vi "TrapezoidalMotionProfile.vi"(6 "Initialize":bool, 10 "Time":dbl, 11 "Config":T2={"TargetPos"=10.0, "InitalPos"=0.0, "FinalVel"=0.0, "IntitialVel"=0.0, "MaxVel"=10.0, "MaxAccel"=10.0}) -> (0 "Done":bool, 2 "Velocity":dbl, 3 "Distance":dbl)   [LabVIEW 2017]
panel:
  out "Data 2":T1
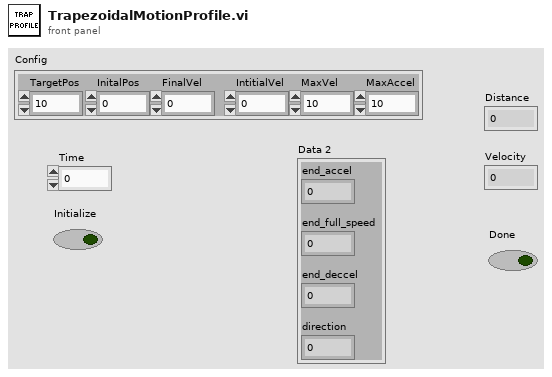
[diagram p1: front panel]
types:
  T1 = cluster{"end_accel":dbl, "end_full_speed":dbl, "end_deccel":dbl, "direction":dbl}
  T2 = cluster{"TargetPos":dbl, "InitalPos":dbl, "FinalVel":dbl, "IntitialVel":dbl, "MaxVel":dbl, "MaxAccel":dbl}
  T3 = cluster{"Config":cluster{"TargetPos":dbl, "InitalPos":dbl, "FinalVel":dbl, "IntitialVel":dbl, "MaxVel":dbl, "MaxAccel":dbl}, "Data 2":cluster{"end_accel":dbl, "end_full_speed":dbl, "end_deccel":dbl, "direction":dbl}}
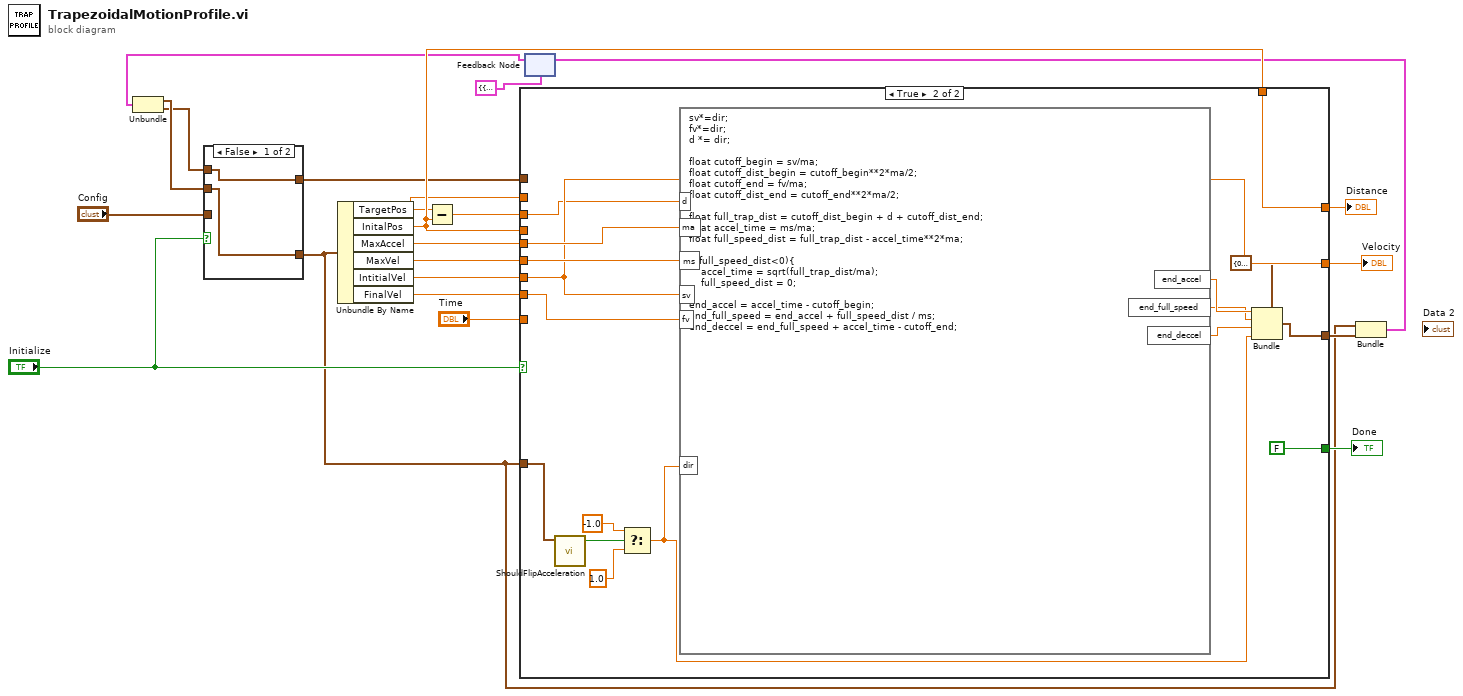
[diagram p0: block diagram]
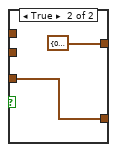
[diagram p2: hidden frame]
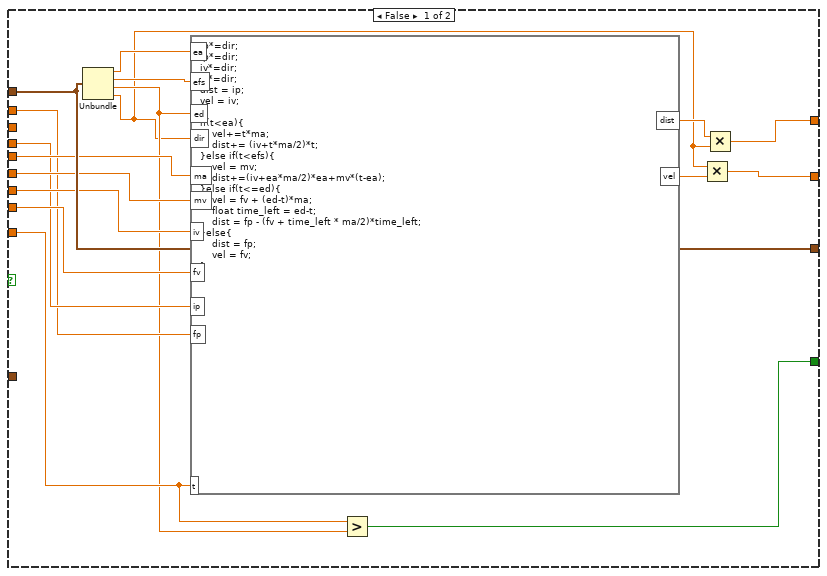
[diagram p3: hidden frame]
diagram:
  n1 = feedback #1(T3 {"Config"={"TargetPos"=10.0, "InitalPos"=0.0, "FinalVel"=0.0, "IntitialVel"=0.0, "MaxVel"=10.0, "MaxAccel"=10.0}, "Data 2"={"end_accel"=0.0, "end_full_speed"=0.0, "end_deccel"=0.0, "direction"=0.0}} ("AllData")) -> (w6:T3)
  n2 = Unbundle(w6) -> ("Config"=w5:T2, "Data 2"=w4:T1)
  n3 = case shown="False" "Initialize" {
    tunnel: [w22 T1 {"end_accel"=0.0, "end_full_speed"=0.0, "end_deccel"=0.0, "direction"=0.0} ("Data 2")] -> w9
    tunnel: [w23 w24] -> w2
    tunnel: "Config" -> [_ w24]
    tunnel: w5 -> [w23 _]
    tunnel: w4 -> [w22 _]
    frame False {
    }
    frame True {
    }
  }
  n4 = Unbundle By Name(w2) -> ("TargetPos"=w11:dbl, "InitalPos"=w12:dbl, "MaxAccel"=w21:dbl, "MaxVel"=w20:dbl, "IntitialVel"=w18:dbl, "FinalVel"=w14:dbl)
  n5 = Subtract(x=w11, y=w12) -> (x-y=w19:dbl)
  n6 = case shown="True" "Initialize" {
    tunnel: w21 -> [w39 w59]
    tunnel: w20 -> [w37 w58]
    tunnel: w18 -> [w38 w56]
    tunnel: w19 -> [_ w48]
    tunnel: [w27 w56] -> w17
    tunnel: [w29 w47] -> w13
    tunnel: w9 -> [w42 _]
    tunnel: [w42 w46] -> w3
    tunnel: "Time" -> [w33 _]
    tunnel: [w31 FALSE ("Initialize")] -> w15
    tunnel: w2 -> [_ w54]
    tunnel: w14 -> [w36 w53]
    tunnel: w12 -> [_ w47]
    tunnel: w12 -> [w35 _]
    tunnel: w11 -> [w34 _]
    frame False {
      n7 = Unbundle(w42) -> ("end_accel"=w41:dbl, "end_full_speed"=w40:dbl, "end_deccel"=w32:dbl, "direction"=w26:dbl)
      n8 = formula code="ip*=dir;\nfp*=dir;\niv*=dir;\nfv*=dir;\ndist = ip;\nvel = iv;\n\nif(t<ea){\n    vel+=t*ma;\n    dist+= (iv+t*ma/2)*t;\n}else if(t<efs){\n    vel = mv;\n    dist+=(iv+ea*ma/2)*ea+mv*(t-ea);\n}else if(t<=ed){\n    vel = fv + (ed-t)*ma;\n    float time_left = ed-t;\n    dist = fp - (fv + time_left * ma/2)*time_left;\n}else{\n    dist = fp;\n    vel = fv;\n}"("t"=w33, "ea"=w41, "efs"=w40, "ed"=w32, "ma"=w39, "iv"=w38, "mv"=w37, "fv"=w36, "ip"=w35, "fp"=w34, "dir"=w26) -> ("dist"=w30:dbl, "vel"=w28:dbl)
      n9 = Greater?(x=w33, y=w32) -> (0:w31:bool)
      n10 = Multiply(x=w26, y=w28) -> (x*y=w27:dbl)
      n11 = Multiply(x=w30, y=w26) -> (x*y=w29:dbl)
    }
    frame True {
      n12 = call "ShouldFlipAcceleration.vi"("Config"=w54) -> ("Flip?"=w51:bool)  [unwired: 10 in]
      n13 = Select(t=-1.0, s=w51, f=1.0) -> (s? t:f=w43:dbl)
      n14 = formula code="sv*=dir;\nfv*=dir;\nd *= dir;\n\nfloat cutoff_begin = sv/ma;\nfloat cutoff_dist_begin = cutoff_begin**2*ma/2;\nfloat cutoff_end = fv/ma;\nfloat cutoff_dist_end = cutoff_end**2*ma/2;\n\nfloat full_trap_dist = cutoff_dist_begin + d + cutoff_dist_end;\nfloat accel_time = ms/ma;\nfloat full_speed_dist = full_trap_dist - accel_time**2*ma;\n\nif(full_speed_dist<0){\n    accel_time = sqrt(full_trap_dist/ma);\n    full_speed_dist = 0;\n}\nend_accel = accel_time - cutoff_begin;\nend_full_speed = end_accel + full_speed_dist / ms;\nend_deccel = end_full_speed + accel_time - cutoff_end;"("ma"=w59, "ms"=w58, "d"=w48, "sv"=w56, "fv"=w53, "dir"=w43) -> ("end_accel"=w57:dbl, "end_full_speed"=w45:dbl, "end_deccel"=w44:dbl)
      n15 = Bundle(cluster=T1 {"end_accel"=0.0, "end_full_speed"=0.0, "end_deccel"=0.0, "direction"=0.0} ("Data 2"), "end_accel"=w57, "end_full_speed"=w45, "end_deccel"=w44, "direction"=w43) -> (w46:T1)
    }
  }
  "Distance" <- w13
  "Velocity" <- w17
  "Done" <- w15
  n16 = Bundle("Config"=w2, "Data 2"=w3) -> (w1:T3)  [unwired: 1 in]
  n17 = feedback-in #1(w1) -> ()
